vi "Do Collision Teams Array.vi"(7 "Teams In":refnum<class "Team.lvclass">[](array[class]), 8 "Team":i32, 11 "Square":refnum<class "Square.lvclass">) -> (5 "Teams out":refnum<class "Team.lvclass">[](array[class]))   [LabVIEW 2020, in "SquareBattle.lvlib" / "Square.lvclass"]
uses:
  Square.lvclass
  Square.lvclass/Square.ctl
  Team/Team.lvclass
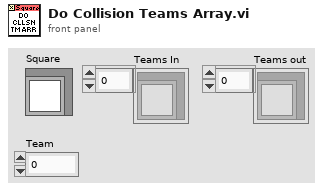
[diagram p1: front panel]
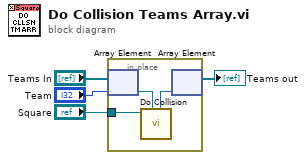
[diagram p0: block diagram]
diagram:
  n1 = in-place {
    in-place-border: "Square" -> [w6]
    n2 = in-place-array #1("Teams In", "Team") -> (w7:refnum<class "Team.lvclass">)
    n3 = call "Do Collision.vi"("Team in"=w7, "Square"=w6) -> ("Team out"=w5:refnum<class "Team.lvclass">)  [unwired: 9 in]
    n4 = in-place-array #1(w5) -> (→"Teams out":refnum<class "Team.lvclass">[])  [unwired: 1 out]
  }
